vi "Tree Column Header.vi"(7 "Action":T1, 8 "error in (no error)":errorcluster, 10 "Class Name":string, 11 "Tree Ref":refnum<vi>) -> (0 "error out":errorcluster, 3 "Tree Column Header":string)   [LabVIEW 2023]
uses:
  controls/action enum.ctl
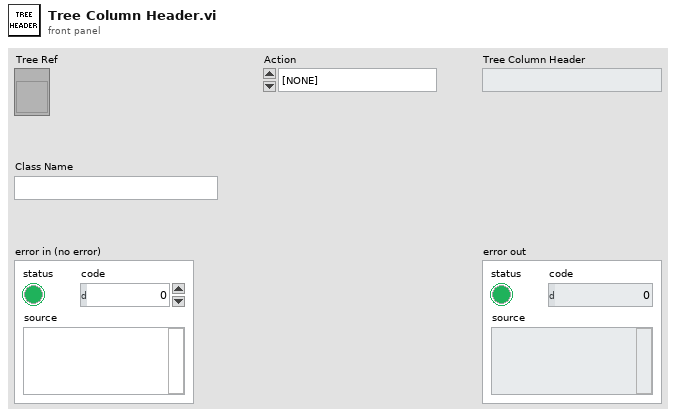
[diagram p1: front panel]
types:
  T1 = typedef "action enum.ctl" = enum16{"[NONE]", "APP_SEPARATOR", "Wire Bundle", "Wire Unbundle", "Terminal Unbundle", "Terminal Bundle", "Bundler Move Up", "Bundler Move Down", "Bundler Insert", "Bundler Remove", "Bundler Remove Unwired", "Bundler Reorder", "In Place Insert", "In Place Remove", "In Place Remove Unwired", "In Place Reorder", "Wire Properties", "Wire Method", "Terminal Properties", "Terminal Method", "Property Move Up", "Property Move Down", "Properties Insert", "Properties Remove", "Properties Remove Unwired", "Properties Reorder", "Method Change", "Class For Constant", "Class For Control", "Class For Node", "Class Name to Clipboard"}
  T2 = enum16{"None", "Cluster", "Property", "Method", "Class"}
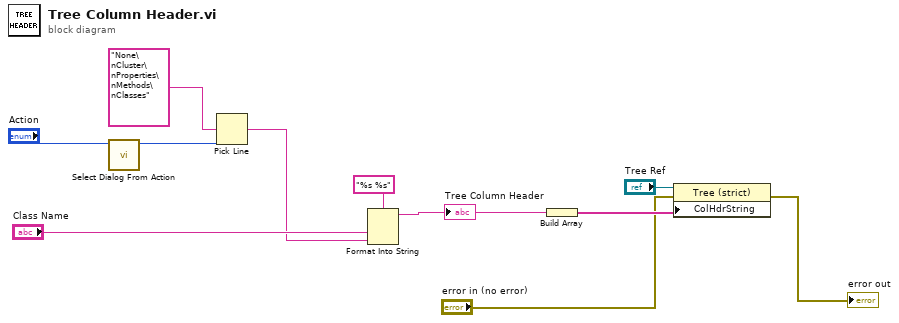
[diagram p0: block diagram]
diagram:
  n1 = call "Select Dialog From Action.vi"("Action"="Action") -> ("Dialog Selection"=w10:T2)  [unwired: 10 in]
  n2 = Pick Line(multi-line string="None\nCluster\nProperties\nMethods\nClasses", line index=w10) -> (output string=w6:string)  [unwired: 1 in]
  n3 = Format Into String(format string="%s %s", "Class Name", w6) -> (resulting string=w4:string)  [unwired: 2 in, 1 out]
  "Tree Column Header" <- w4
  n4 = Build Array(w4) -> (w3:string[])
  n5 = property class="Tree (strict)"(reference="Tree Ref", error in="error in (no error)", "ColHdrString"=w3) -> (error out=→"error out":errorcluster)  [unwired: 1 out]
